vi "BuildXYGraph.vi"(1 "y scale 2":dbl, 2 "y scale 1":dbl, 3 "xscale":dbl, 4 "Old Graph":cluster{"Y":dbl[], "Y":dbl[]}[](array[cluster])) -> (0 "New Graph":cluster{"Y":dbl[], "Y":dbl[]}[](array[cluster]))   [LabVIEW 2016]
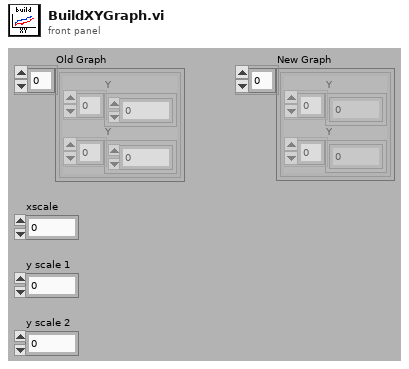
[diagram p1: front panel]
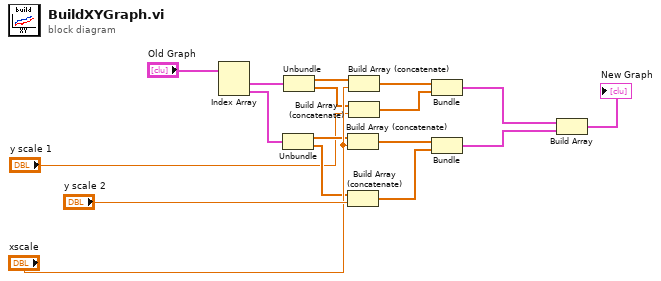
[diagram p0: block diagram]
diagram:
  n1 = Index Array(array="Old Graph") -> (element #1=w8:cluster{"Y":dbl[], "Y":dbl[]}, element #2=w16:cluster{"Y":dbl[], "Y":dbl[]})  [unwired: 2 in]
  n2 = Unbundle(w16) -> ("Y"=w12:dbl[], "Y"=w13:dbl[])
  n3 = Unbundle(w8) -> ("Y"=w9:dbl[], "Y"=w10:dbl[])
  n4 = Build Array (concatenate)(w12, "xscale") -> (w5:dbl[])
  n5 = Build Array (concatenate)(w13, "y scale 2") -> (w3:dbl[])
  n6 = Build Array (concatenate)(w9, "xscale") -> (w6:dbl[])
  n7 = Build Array (concatenate)(w10, "y scale 1") -> (w4:dbl[])
  n8 = Bundle(w6, w4) -> (w1:cluster{dbl[], dbl[]})  [unwired: 1 out]
  n9 = Bundle(w5, w3) -> (w2:cluster{dbl[], dbl[]})  [unwired: 1 out]
  n10 = Build Array(w1, w2) -> (→"New Graph":cluster{dbl[], dbl[]}[])
